vi "vi time get.vi"() -> ()   [LabVIEW 2019, in "test.lvlib"]
uses:
  SubVI/test.lvlib
panel:
  out "Temperature":dbl format="%.2f"
  out "x-y":dbl
  in  "VISA session":refnum<visa-resource-name>
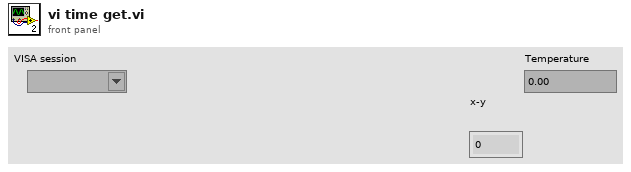
[diagram p1: front panel]
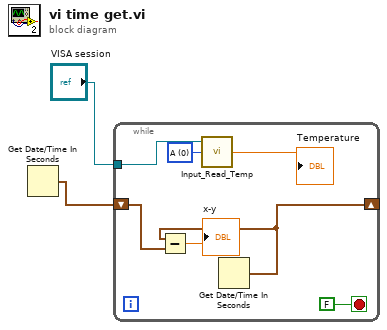
[diagram p0: block diagram]
diagram:
  n1 = Get Date/Time In Seconds() -> (seconds since 1Jan1904=w2:timestamp)
  n2 = while {
    shift-right: [w8] -> _
    shift-left: w2 -> [w7]
    tunnel: "VISA session" -> [w5]
    stop <- FALSE stop-if-true
    w4 = u8 0 items=["A", "B", "C", "D"] ("Input")
    n3 = call "Input_Read_Temp.vi"("Input"=w4, "VISA In"=w5) -> ("Temperature"=→"Temperature":dbl)  [unwired: 1 in, 2 out]
    n4 = Get Date/Time In Seconds() -> (seconds since 1Jan1904=w8:timestamp)
    n5 = Subtract(x=w8, y=w7) -> (x-y=→"x-y":dbl)
  }
